vi "send_to_main.vi"(8 "error in (no error)":errorcluster, 11 "Main state cluster":cluster{"State Enum":T1, "variant":variant}) -> (0 "error out":errorcluster)   [LabVIEW 2010]
uses:
  typedefs/main_state_enum.ctl
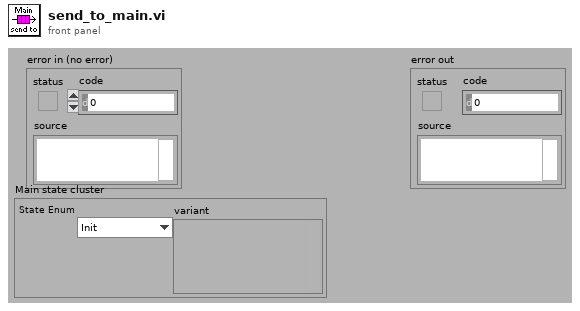
[diagram p1: front panel]
types:
  T1 = typedef "main_state_enum.ctl" = enum16{"Init", "Empty", "ParamsChanged", "Start", "Stop", "Abort", "Acquisition finished", "SetShutter", "Reset", "Error", "Quit"}
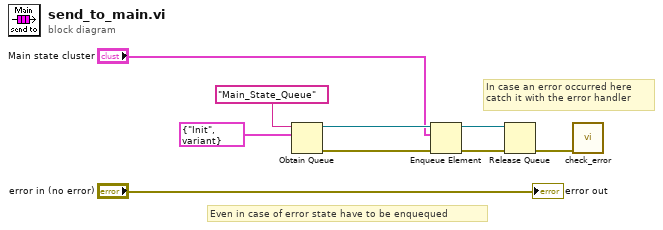
[diagram p0: block diagram]
diagram:
  # "In case an error occurred here\ncatch it with the error handler"
  # "Even in case of error state have to be enquequed"
  n1 = Obtain Queue(name (unnamed)="Main_State_Queue", element data type=cluster{"State Enum":T1, "variant":variant} {"State Enum"=enum."Init", "variant"=variant}) -> (queue out=w6:refnum<queue>, error out=w7:errorcluster)  [unwired: 3 in, 1 out]
  n2 = Enqueue Element(queue=w6, element="Main state cluster", error in (no error)=w7) -> (queue out=w2:refnum<queue>, error out=w4:errorcluster)  [unwired: 1 in, 1 out]
  n3 = Release Queue(queue=w2, error in (no error)=w4) -> (error out=w3:errorcluster)  [unwired: 1 in, 2 out]
  n4 = call "check_error.vi"("error in"=w3) -> ()  [unwired: 10 in, 1 out]
  "error out" <- "error in (no error)"
